vi "FPGA_controller.vi"() -> ()   [LabVIEW 2017]
uses:
  <vilib>/rvi/Emulation/niFpgaGetClockAttributes.vi
  <vilib>/rvi/Emulation/niFpgaSctlEmulationGetInTimedLoop.vi
  <vilib>/rvi/Emulation/niFpgaEmulationReportErrorSimple.vi
  <vilib>/rvi/eio/common/nirviEmuTemplateMethod_errors.vi
  <vilib>/rvi/Emulation/niFpgaCriticalErrorInLSC.vi
  <vilib>/eio/EIONode/EIONode.xnode
panel:
  out "Translated":i16
  out "VALID":bool
  in  "Scale x2":fxp<+/-,32,16>=10.0 format="%#_21g"
  in  "m_first x2":fxp<+/-,49,33>=4.9499969482421875 format="%#_26g"
  in  "Offset x2":fxp<+/-,48,32> format="%#_26g"
  in  "1/eta x":fxp<+/-,32,16>=200.0 format="%#_21g"
  in  "m_first x1":fxp<+/-,49,33>=0.649993896484375 format="%#_26g"
  in  "Offset x1":fxp<+/-,48,32> format="%#_26g"
  in  "Scale x1":fxp<+/-,32,16>=5.0 format="%#_21g"
  in  "stop":bool
  # "STATES CONVERSION"
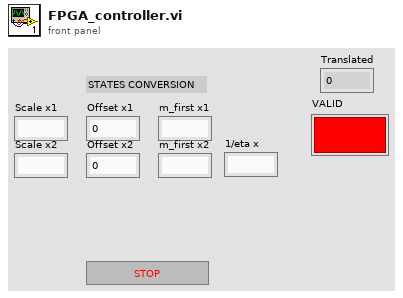
[diagram p1: front panel]
types:
  T1 = cluster{"Boolean array[0]":bool, "Boolean array[1]":bool, "Boolean array[2]":bool, "Boolean array[3]":bool, "Boolean array[4]":bool, "Boolean array[5]":bool, "Boolean array[6]":bool, "Boolean array[7]":bool, "Boolean array[8]":bool, "Boolean array[9]":bool, "Boolean array[10]":bool, "Boolean array[11]":bool, "Boolean array[12]":bool, "Boolean array[13]":bool, "Boolean array[14]":bool, "Boolean array[15]":bool}
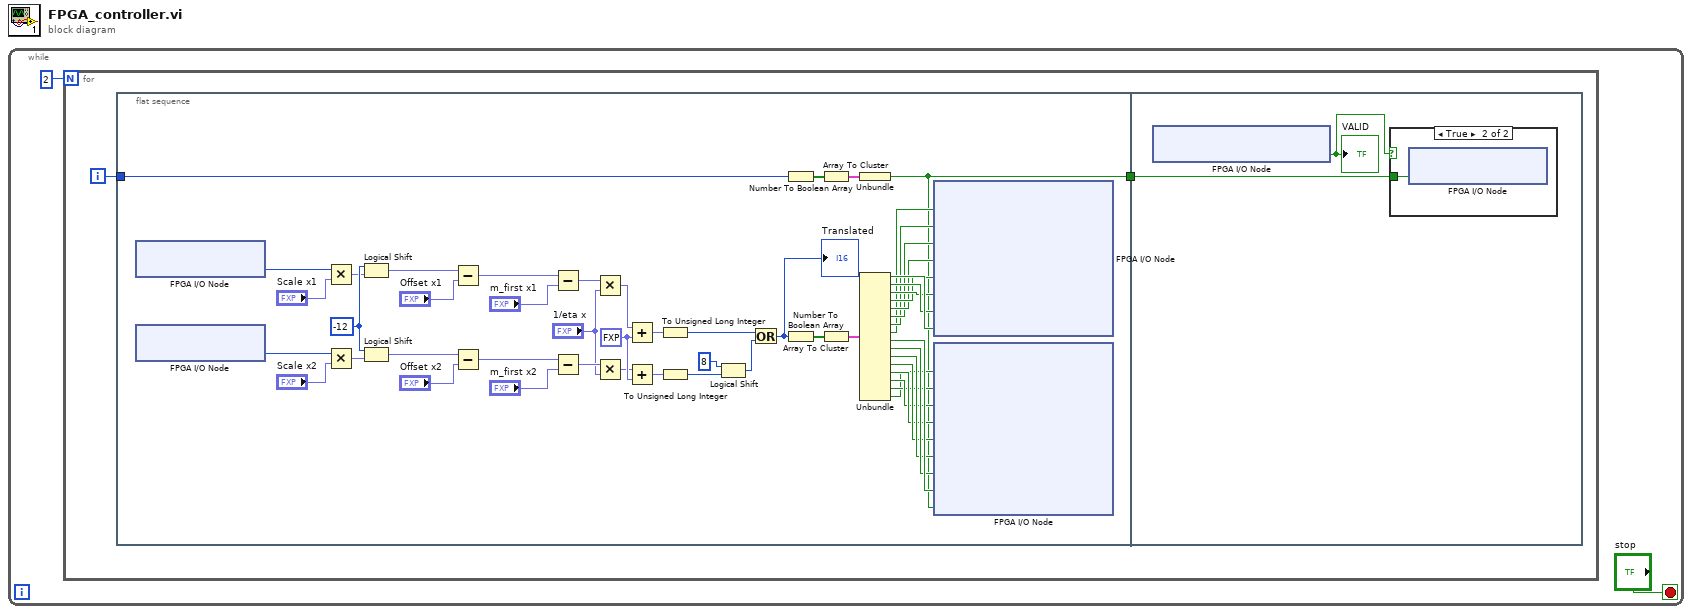
[diagram p0: block diagram]
diagram:
  n1 = while {
    stop <- "stop" stop-if-true
    n2 = for {
      N: 2 -> [_]
      i -> [w4]
      n3 = flat-sequence {
        tunnel: w4 -> [w35]
        tunnel: [w33] -> w3
        tunnel: w3 -> [w56]
        frame #0 {
          w28 = fxp<+/-,64,32> 0.5 ("y")
          w26 = i16 -12 ("y")
          n4 = xnode "FPGA I/O Node"() -> ("ConnectorA/AI0"=w16:u16)  [unwired: 1 in, 1 out]
          n5 = xnode "FPGA I/O Node"() -> ("ConnectorA/AI1"=w15:u16)  [unwired: 1 in, 1 out]
          n6 = Multiply(x=w16, y="Scale x1") -> (x*y=w25:fxp<+/-,48,32>)
          n7 = Multiply(x=w15, y="Scale x2") -> (x*y=w29:fxp<+/-,48,32>)
          n8 = Logical Shift(y=w26, x=w25) -> (x << y=w22:fxp<+/-,48,32>)
          n9 = Logical Shift(y=w26, x=w29) -> (x << y=w19:fxp<+/-,48,32>)
          n10 = Subtract(x=w22, y="Offset x1") -> (x-y=w23:fxp<+/-,49,33>)
          n11 = Subtract(x=w19, y="Offset x2") -> (x-y=w20:fxp<+/-,49,33>)
          n12 = Subtract(x=w23, y="m_first x1") -> (x-y=w24:fxp<+/-,50,34>)
          n13 = Subtract(x=w20, y="m_first x2") -> (x-y=w18:fxp<+/-,50,34>)
          n14 = Multiply(x=w24, y="1/eta x") -> (x*y=w21:fxp<+/-,64,49>)
          n15 = Multiply(x=w18, y="1/eta x") -> (x*y=w17:fxp<+/-,64,49>)
          n16 = Add(x=w21, y=w28) -> (x+y=w32:fxp<+/-,64,50>)
          n17 = Add(x=w17, y=w28) -> (x+y=w27:fxp<+/-,64,50>)
          n18 = To Unsigned Long Integer(number=w32) -> (unsigned 32bit integer=w7:u32)
          n19 = To Unsigned Long Integer(number=w27) -> (unsigned 32bit integer=w30:u32)
          n20 = Logical Shift(y=8, x=w30) -> (x << y=w6:u32)
          n21 = Or(x=w7, y=w6) -> (x .or. y?=w5:u32)
          "Translated" <- w5
          n22 = Number To Boolean Array(number=w35) -> (Boolean array=w36:bool[])
          n23 = Number To Boolean Array(number=w5) -> (Boolean array=w53:bool[])
          n24 = Array To Cluster(array=w36) -> (cluster=w34:cluster{"Boolean array[0]":bool})
          n25 = Array To Cluster(array=w53) -> (cluster=w54:T1)
          n26 = Unbundle(w34) -> ("Boolean array[0]"=w33:bool)
          n27 = Unbundle(w54) -> ("Boolean array[0]"=w52:bool, "Boolean array[1]"=w51:bool, "Boolean array[2]"=w50:bool, "Boolean array[3]"=w49:bool, "Boolean array[4]"=w48:bool, "Boolean array[5]"=w47:bool, "Boolean array[6]"=w46:bool, "Boolean array[7]"=w45:bool, "Boolean array[8]"=w44:bool, "Boolean array[9]"=w43:bool, "Boolean array[10]"=w42:bool, "Boolean array[11]"=w41:bool, "Boolean array[12]"=w40:bool, "Boolean array[13]"=w39:bool, "Boolean array[14]"=w38:bool, "Boolean array[15]"=w37:bool)
          n28 = xnode "FPGA I/O Node"("Component-Level IP\\pi00"=w45, "Component-Level IP\\pi01"=w46, "Component-Level IP\\pi02"=w47, "Component-Level IP\\pi03"=w48, "Component-Level IP\\pi04"=w49, "Component-Level IP\\pi05"=w50, "Component-Level IP\\pi06"=w51, "Component-Level IP\\pi07"=w52) -> ()  [unwired: 8 in, 8 out]
          n29 = xnode "FPGA I/O Node"("Component-Level IP\\pi08"=w37, "Component-Level IP\\pi09"=w38, "Component-Level IP\\pi10"=w39, "Component-Level IP\\pi11"=w40, "Component-Level IP\\pi12"=w41, "Component-Level IP\\pi13"=w42, "Component-Level IP\\pi14"=w43, "Component-Level IP\\pi15"=w44, "Component-Level IP\\pi16"=w33) -> ()  [unwired: 9 in, 9 out]
        }
        frame #1 {
          n30 = xnode "FPGA I/O Node"() -> ("Component-Level IP\\po0"=w55:bool)  [unwired: 1 in, 1 out]
          "VALID" <- w55
          n31 = case shown="True" w55 {
            tunnel: w56 -> [_ w57]
            frame False {
            }
            frame True {
              n32 = xnode "FPGA I/O Node"("ConnectorA/DIO0"=w57) -> ()  [unwired: 1 in, 1 out]
            }
          }
        }
      }
    }
  }
